vi "SDT_ReadFile.vi"(8 "error in":errorcluster, 11 "sdtFile":path=path "X:/FQ/ExampleFiles/Mushrooms/agaricus-04-big.sdt") -> (0 "error out":errorcluster, 1 "MeasureInfo":T7[](array[typedef]) {"MeasFCSInfo"."fcs_decay_calc" format="%x"; "MeasStopInfo"."flags" format="x%x"; "MeasureInfo_PartB"."mod_type2" format="%016x"; "MeasureInfo_PartB"."mod_type1" format="%016x"; "MeasureInfo_PartB"."tac_r" format="%^#_4g"}, 2 "SumOfDecays":dbl[][](graph), 3 "IntensityImage":cluster{"Intensity Graph":u8[][]}[](array[cluster]), 4 "DecayMatrix":cluster{"Waveform Graph":sgl[]}[][](array[cluster]), 5 "SPCdata":T1[](array[typedef]), 6 "SetUp":string, 7 "ActiveModule":string[](array[string]))   [LabVIEW 2023]
doc: "This VI reads a SDT-file from disc. The header and block data is interpreted and displayed. The usage and information in the graphs depends on the type of data stored in the SDT-file.\nFor a description of the *.sdt file format see: SPC_data_file_structure.h\nUse this VI to display data stored previously in a SDT-file or to create your own analysis on this data. \n\ninfo@becker-hickl.com"
uses:
  SPC_Wrappers/SPC_Controls/bhfile_header.ctl
  SPC_Wrappers/SPC_Controls/BHModuleType.ctl
  SPC_Wrappers/SPC_Controls/MeasureInfo.ctl
  SPC_Wrappers/SPC_Controls/MeasureInfo_PartB.ctl
  SPC_Wrappers/SPC_Controls/MeasStopInfo.ctl
  SPC_Wrappers/SPC_Controls/MeasFCSInfo.ctl
  SPC_Wrappers/SPC_Controls/MeasureInfo_PartE.ctl
  SPC_Wrappers/SPC_Controls/MeasHISTInfo.ctl
  SPC_Wrappers/SPC_Controls/HISTInfoExt.ctl
  SPC_Wrappers/SPC_Controls/MeasureInfo_PartI.ctl
  SPC_Wrappers/SPC_Controls/MeasureInfo_PartK.ctl
  SPC_Wrappers/SPC_Controls/MeasureInfo_PartM.ctl
  SPC_Wrappers/SPC_Controls/BHFileBlockHeader_interpreted.ctl
  SPC_Wrappers/SPC_Controls/BHFileBlockHeader.ctl
  SPC_Wrappers/SPC_Controls/BlockType_DataType.ctl
  SPC_Wrappers/SPC_Controls/BlockType_Contents.ctl
  SPC_Wrappers/SPC_Controls/BlockType_CreationMode.ctl
  SPC_Wrappers/SPC_Controls/SPCdata.ctl
panel:
  out "mod_type":string[](array[string])
  out "BHFileBlockHeader_interpreted":T2[](array[typedef]) {"lblock_RoutingCh" format="%.0x"; "BlockNo" format="%.0x"; "lblock_Contents" items=["DECAY_BLOCK"=0, "PAGE_BLOCK"=16, "FCS_BLOCK"=32, "FIDA_BLOCK"=48, "FILDA_BLOCK"=64, "MCS_BLOCK"=80, "IMG_BLOCK"=96, "MCST_BLOCK"=112, "IMG_MCS_BLOCK"=128, "MOM_BLOCK"=144, "IMG_INT_BLOCK"=160, "IMG_WF_BLOCK"=176, "IMG_LIFE_BLOCK"=192]; "CreationMode" items=["NOT_USED"=0, "MEAS_DATA"=1, "FLOW_DATA"=2, "MEAS_DATA_FROM_FILE"=3, "CALC_DATA"=4, "SIM_DATA"=5, "FIFO_DATA"=8, "FIFO_DATA_FROM_FILE"=9, "MOM_DATA"=10, "MOM_DATA_FROM_FILE"=11]; "Contents" items=["DECAY_BLOCK"=0, "PAGE_BLOCK"=16, "FCS_BLOCK"=32, "FIDA_BLOCK"=48, "FILDA_BLOCK"=64, "MCS_BLOCK"=80, "IMG_BLOCK"=96, "MCST_BLOCK"=112, "IMG_MCS_BLOCK"=128, "MOM_BLOCK"=144, "IMG_INT_BLOCK"=160, "IMG_WF_BLOCK"=176, "IMG_LIFE_BLOCK"=192]; "DataType" items=["DATA_USHORT (U16)"=0, "DATA_ULONG (U32)"=256, "DATA_DBL (DBL64)"=512]; "BHFileBlockHeader"."lblock_no" format="x%x"; "BHFileBlockHeader"."block_type" format="%x"}
  out "SetUpLength":i32
  out "MagicNum":u16 format="%x"
  out "FCS_Block":cluster{"XY Graph":cluster{dbl[], dbl[]}}[](array[cluster])
  out "BinarySetup_length":u16
  out "ModuleSubtype":i16
  out "BHModuleType":T17=32 format="x%x" items=["SPC-130"=32, "SPC-600"=33, "SPC-630"=34, "SPC-700"=35, "SPC-730"=36, "SPC-830"=37, "SPC-140"=38, "SPC-930"=39, "SPC-150"=40, "DPC-230"=41, "SPC-130EM"=42, "SPC-160"=43, "SPC-150N"=46, "PMS-800"=51, "SPC-150NX"=128, "SPC-160X"=129, "SPC-160PCIE"=130, "SPC-130EMN"=131, "SPC-180N"=132, "SPC-180NX"=133, "SPC-180NXX"=134, "SPC-180N-USB"=135, "SPC-130IN"=136, "SPC-130INX"=137, "SPC-130INXX"=138, "SPC-QC-104"=139, "Simulation"=-1]
  out "SoftwareRevision":i16
  out "FileInfo":string
  out "bhfile_header":T18 {"chksum" format="x%x"; "header_valid" format="x%x"}
  # "block_type"
  # "lblock_no"
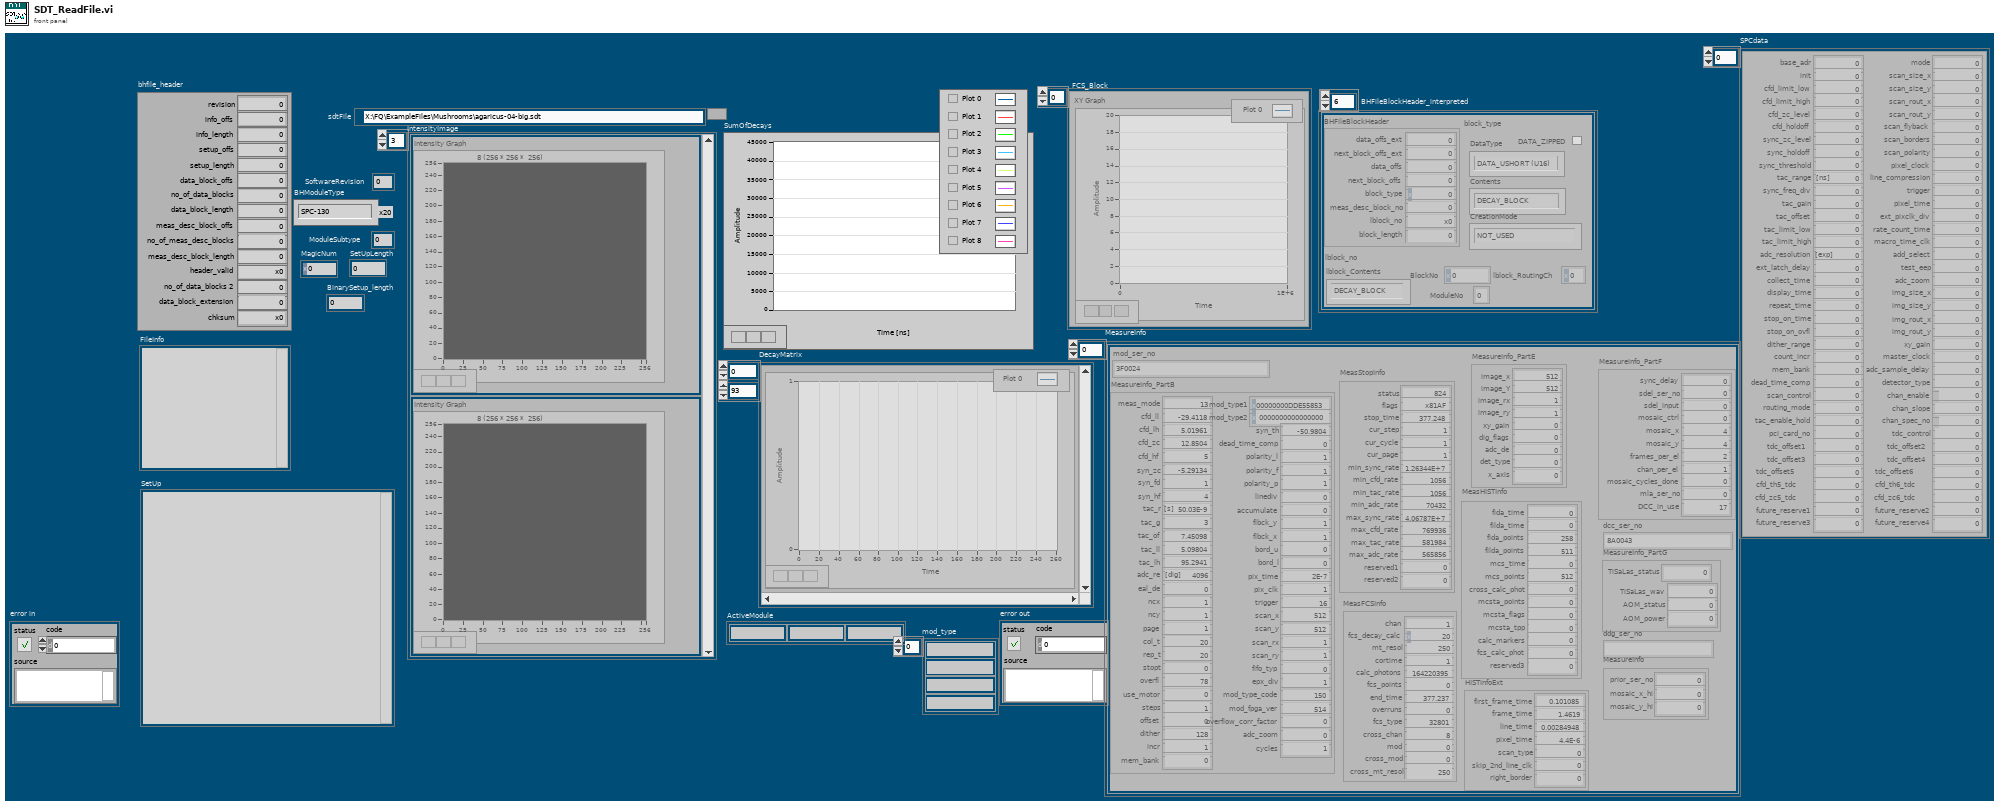
[diagram p1: front panel]
types:
  T1 = typedef "SPCdata.ctl" = cluster{"base_adr":u16, "init":i16, "cfd_limit_low":sgl, "cfd_limit_high":sgl, "cfd_zc_level":sgl, "cfd_holdoff":sgl, "sync_zc_level":sgl, "sync_holdoff":sgl, "sync_threshold":sgl, "tac_range":sgl, "sync_freq_div":i16, "tac_gain":i16, "tac_offset":sgl, "tac_limit_low":sgl, "tac_limit_high":sgl, "adc_resolution":i16, "ext_latch_delay":i16, "collect_time":sgl, "display_time":sgl, "repeat_time":sgl, "stop_on_time":i16, "stop_on_ovfl":i16, "dither_range":i16, "count_incr":i16, "mem_bank":i16, "dead_time_comp":i16, "scan_control":u16, "routing_mode":u16, "tac_enable_hold":sgl, "pci_card_no":i16, "mode":u16, "scan_size_x":u32, "scan_size_y":u32, "scan_rout_x":u32, "scan_rout_y":u32, "scan_flyback":u32, "scan_borders":u32, "scan_polarity":u16, "pixel_clock":u16, "line_compression":u16, "trigger":u16, "pixel_time":sgl, "ext_pixclk_div":u32, "rate_count_time":sgl, "macro_time_clk":i16, "add_select":i16, "test_eep":i16, "adc_zoom":i16, "img_size_x":u32, "img_size_y":u32, "img_rout_x":u32, "img_rout_y":u32, "xy_gain":i16, "master_clock":i16, "adc_sample_delay":i16, "detector_type":i16, "chan_enable":u32, "chan_slope":u32, "chan_spec_no":u32, "tdc_control":u32, "tdc_offset1":sgl, "tdc_offset2":sgl, "tdc_offset3":sgl, "tdc_offset4":sgl, "tdc_offset5":sgl, "tdc_offset6":sgl, "cfd_th5_tdc":sgl, "cfd_th6_tdc":sgl, "cfd_zc5_tdc":sgl, "cfd_zc6_tdc":sgl, "future_reserve1":u64, "future_reserve2":u64, "future_reserve3":u64, "future_reserve4":u64}
  T2 = typedef "BHFileBlockHeader_interpreted.ctl" = cluster{"BHFileBlockHeader":T3, "DATA_ZIPPED":bool, "DataType":T4, "Contents":T5, "CreationMode":T6, "lblock_Contents":T5, "ModuleNo":u8, "BlockNo":u32, "lblock_RoutingCh":u32}
  T3 = typedef "BHFileBlockHeader.ctl" = cluster{"data_offs_ext":u8, "next_block_offs_ext":u8, "data_offs":u32, "next_block_offs":u32, "block_type":u16, "meas_desc_block_no":i16, "lblock_no":u32, "block_length":u32}
  T4 = typedef "BlockType_DataType.ctl" = u16
  T5 = typedef "BlockType_Contents.ctl" = u16
  T6 = typedef "BlockType_CreationMode.ctl" = u16
  T7 = typedef "MeasureInfo.ctl" = cluster{"mod_ser_no":string, "MeasureInfo_PartB":T8, "MeasStopInfo":T9, "MeasFCSInfo":T10, "MeasureInfo_PartE":T11, "MeasHISTInfo":T12, "HISTInfoExt":T13, "MeasureInfo_PartF":T14, "dcc_ser_no":string, "MeasureInfo_PartG":T15, "ddg_ser_no":string, "MeasureInfo":T16}
  T8 = typedef "MeasureInfo_PartB.ctl" = cluster{"meas_mode":i16, "cfd_ll":sgl, "cfd_lh":sgl, "cfd_zc":sgl, "cfd_hf":sgl, "syn_zc":sgl, "syn_fd":i16, "syn_hf":sgl, "tac_r":sgl, "tac_g":i16, "tac_of":sgl, "tac_ll":sgl, "tac_lh":sgl, "adc_re":i16, "eal_de":i16, "ncx":i16, "ncy":i16, "page":u16, "col_t":sgl, "rep_t":sgl, "stopt":i16, "overfl":i8, "use_motor":i16, "steps":u16, "offset":sgl, "dither":i16, "incr":i16, "mem_bank":i16, "mod_type1":u64, "mod_type2":u64, "syn_th":sgl, "dead_time_comp":i16, "polarity_l":i16, "polarity_f":i16, "polarity_p":i16, "linediv":i16, "accumulate":i16, "flbck_y":i32, "flbck_x":i32, "bord_u":i32, "bord_l":i32, "pix_time":sgl, "pix_clk":i16, "trigger":i16, "scan_x":i32, "scan_y":i32, "scan_rx":i32, "scan_ry":i32, "fifo_typ":i16, "epx_div":i32, "mod_type_code":u16, "mod_fpga_ver":u16, "overflow_corr_factor":sgl, "adc_zoom":i32, "cycles":i32}
  T9 = typedef "MeasStopInfo.ctl" = cluster{"status":u16, "flags":u16, "stop_time":sgl, "cur_step":i32, "cur_cycle":i32, "cur_page":i32, "min_sync_rate":sgl, "min_cfd_rate":sgl, "min_tac_rate":sgl, "min_adc_rate":sgl, "max_sync_rate":sgl, "max_cfd_rate":sgl, "max_tac_rate":sgl, "max_adc_rate":sgl, "reserved1":i32, "reserved2":sgl}
  T10 = typedef "MeasFCSInfo.ctl" = cluster{"chan":u16, "fcs_decay_calc":u16, "mt_resol":u32, "cortime":sgl, "calc_photons":u32, "fcs_points":i32, "end_time":sgl, "overruns":u16, "fcs_type":u16, "cross_chan":u16, "mod":u16, "cross_mod":u16, "cross_mt_resol":u32}
  T11 = typedef "MeasureInfo_PartE.ctl" = cluster{"image_x":i32, "image_Y":i32, "image_rx":i32, "image_ry":i32, "xy_gain":i16, "dig_flags":i16, "adc_de":i16, "det_type":i16, "x_axis":i16}
  T12 = typedef "MeasHISTInfo.ctl" = cluster{"fida_time":sgl, "filda_time":sgl, "fida_points":i32, "filda_points":i32, "mcs_time":sgl, "mcs_points":i32, "cross_calc_phot":u32, "mcsta_points":u16, "mcsta_flags":u16, "mcsta_tpp":u32, "calc_markers":u32, "fcs_calc_phot":u32, "reserved3":u32}
  T13 = typedef "HISTInfoExt.ctl" = cluster{"first_frame_time":sgl, "frame_time":sgl, "line_time":sgl, "pixel_time":sgl, "scan_type":i16, "skip_2nd_line_clk":i16, "right_border":u32}
  T14 = typedef "MeasureInfo_PartI.ctl" = cluster{"sync_delay":sgl, "sdel_ser_no":u16, "sdel_input":i8, "mosaic_ctrl":i8, "mosaic_x":u8, "mosaic_y":u8, "frames_per_el":i16, "chan_per_el":i16, "mosaic_cycles_done":i32, "mla_ser_no":u16, "DCC_in_use":u8}
  T15 = typedef "MeasureInfo_PartK.ctl" = cluster{"TiSaLas_status":u16, "TiSaLas_wav":u16, "AOM_status":u8, "AOM_power":u8}
  T16 = typedef "MeasureInfo_PartM.ctl" = cluster{"prior_ser_no":i32, "mosaic_x_hi":u8, "mosaic_y_hi":u8}
  T17 = typedef "BHModuleType.ctl" = i16
  T18 = typedef "bhfile_header.ctl" = cluster{"revision":i16, "info_offs":i32, "info_length":i16, "setup_offs":i32, "setup_length":u16, "data_block_offs":i32, "no_of_data_blocks":i16, "data_block_length":u32, "meas_desc_block_offs":i32, "no_of_meas_desc_blocks":i16, "meas_desc_block_length":i16, "header_valid":u16, "no_of_data_blocks 2":u32, "data_block_extension":u16, "chksum":u16}
  T19 = enum16{"big-endian, network order", "native, host order", "little-endian"}
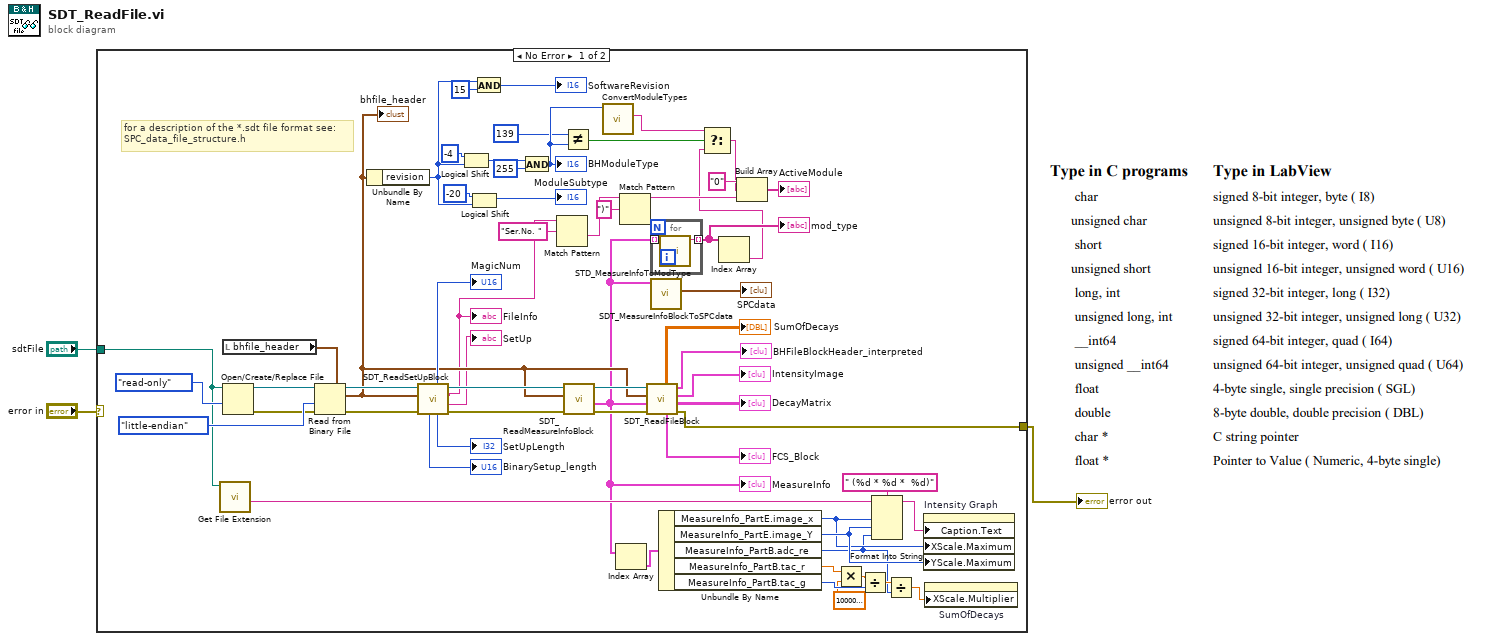
[diagram p0: block diagram]
diagram:
  n1 = case shown="No Error" "error in" {
    selector: "error in" -> [_ w66]
    tunnel: "sdtFile" -> [w23 _]
    tunnel: [w22 w66] -> w1
    frame No Error {
      # "for a description of the *.sdt file format see:\nSPC_data_file_structure.h"
      n2 = call <vilib>:"Get File Extension.vi"("file"=w23) -> ("filename without extension"=w56:string)  [unwired: 6 in, 4 out]
      n3 = local read "bhfile_header"() -> (w44:T18)
      n4 = Open/Create/Replace File(file path (use dialog)=w23, access (0:read/write)=enum16{"read/write", "read-only", "write-only"}."read-only") -> (refnum out=w52:refnum<file>, error out=w4:errorcluster)  [unwired: 4 in, 1 out]
      n5 = Read from Binary File(5:w44, 8:w4, 9:T19."little-endian" ("byte order (0:big-endian, network order)"), 11:w52) -> (0:w43:errorcluster, 2:w35:T18, 3:w50:refnum<file>)  [unwired: 2 in, 1 out]
      "bhfile_header" <- w35
      n6 = Unbundle By Name(w35) -> ("revision"=w51:i16)
      n7 = call "SDT_ReadSetUpBlock.vi"("error in"=w43, "bhfile_header"=w35, "SDTFileRefnum"=w50) -> ("error out"=w42:errorcluster, "SetUp"=→"SetUp":string, "FileInfo"=w15:string, "SDTFileRefnum"=w49:refnum<file>, "SetUpLength"=→"SetUpLength":i32, "MagicNum"=→"MagicNum":u16, "BinarySetup_length"=→"BinarySetup_length":u16)  [unwired: 1 in, 1 out]
      "FileInfo" <- w15
      n8 = Logical Shift(y=i16 -4, x=w51) -> (x << y=w60:i16)
      n9 = Logical Shift(y=i16 -20, x=w51) -> (x << y=→"ModuleSubtype":i16)
      n10 = And(x=w51, y=i16 15) -> (x .and. y?=→"SoftwareRevision":i16)
      n11 = And(x=w60, y=i16 255) -> (x .and. y?=w12:i16)
      "BHModuleType" <- w12
      n12 = Match Pattern(string=w15, regular expression="Ser.No. ") -> (after substring=w20:string)  [unwired: 1 in, 3 out]
      n13 = Not Equal?(x=i16 139 ("y"), y=w12) -> (x != y?=w10:bool)
      n14 = call "SDT_ReadMeasureInfoBlock.vi"("error in"=w42, "bhfile_header"=w35, "SDTFileRefnum"=w49) -> ("error out"=w34:errorcluster, "MeasureInfo"=w7:T7[], "SDTFileRefnum"=w36:refnum<file>)  [unwired: 6 in]
      "MeasureInfo" <- w7
      n15 = call "ConvertModuleTypes.vi"("BHModuleType"=w12) -> ("ModuleTypeString"=w9:string)  [unwired: 8 in, 2 out]
      n16 = Index Array(array=w7) -> (element=w13:T7)  [unwired: 1 in]
      n17 = Match Pattern(string=w20, regular expression=")") -> (before substring=w18:string)  [unwired: 1 in, 3 out]
      n18 = call "SDT_ReadFileBlock.vi"("error in"=w34, "MeasureInfo"=w7, "bhfile_header"=w35, "SDTFileRefnum"=w36) -> ("error out"=w22:errorcluster, "DecayMatrix"=→"DecayMatrix":cluster{"Waveform Graph":sgl[]}[][], "IntensityImage"=→"IntensityImage":cluster{"Intensity Graph":u8[][]}[], "BHFileBlockHeader_interpreted"=→"BHFileBlockHeader_interpreted":T2[], "FCS_Block"=→"FCS_Block":cluster{"XY Graph":cluster{dbl[], dbl[]}}[], "SumOfDecays"=→"SumOfDecays":dbl[][])  [unwired: 2 in]
      n19 = for {
        tunnel: w7 -> [w65] mode=indexing
        tunnel: [w64] -> w6 mode=indexing
        n20 = call "STD_MeasureInfoToModType.vi"("MeasureInfo"=w65) -> ("mod_type"=w64:string)  [unwired: 10 in]
      }
      "mod_type" <- w6
      n21 = call "SDT_MeasureInfoBlockToSPCdata.vi"("MeasureInfo"=w7) -> ("SPCdata"=→"SPCdata":T1[])  [unwired: 10 in]
      n22 = Unbundle By Name(w13) -> ("MeasureInfo_PartE.image_x"=w40:i32, "MeasureInfo_PartE.image_Y"=w41:i32, "MeasureInfo_PartB.adc_re"=w27:i16, "MeasureInfo_PartB.tac_r"=w31:sgl, "MeasureInfo_PartB.tac_g"=w30:i16)
      n23 = Index Array(array=w6) -> (element=w5:string)  [unwired: 1 in]
      n24 = Select(t=w9, s=w10, f=w5) -> (s? t:f=w8:string)
      n25 = Build Array("0" ("element"), w8, w18) -> (→"ActiveModule":string[])
      n26 = Multiply(x=w31, y=sgl 1000000000.0 ("x")) -> (x*y=w26:sgl)
      n27 = Divide(x=w26, y=w30) -> (x/y=w29:sgl)
      n28 = Format Into String(format string=" (%d * %d *  %d)", initial string=w56, w40, w41, w27) -> (resulting string=w54:string)  [unwired: 1 in, 1 out]
      n29 = Divide(x=w29, y=w27) -> (x/y=w28:sgl)
      n30 = property on="Intensity Graph" class="IntGraph (strict)"("Caption.Text"=w54, "XScale.Maximum"=w40, "YScale.Maximum"=w41) -> ()  [unwired: 2 in, 2 out]
      n31 = property on="SumOfDecays" class="WFGraph (strict)"("XScale.Multiplier"=w28) -> ()  [unwired: 2 in, 2 out]
    }
    frame Error {
    }
  }
  "error out" <- w1
